vi "Get Model Construction - with check.vi"(1 "panel record":string[](array[string])) -> (0 "Fabric Array":string[][](array[string]))   [LabVIEW 2010]
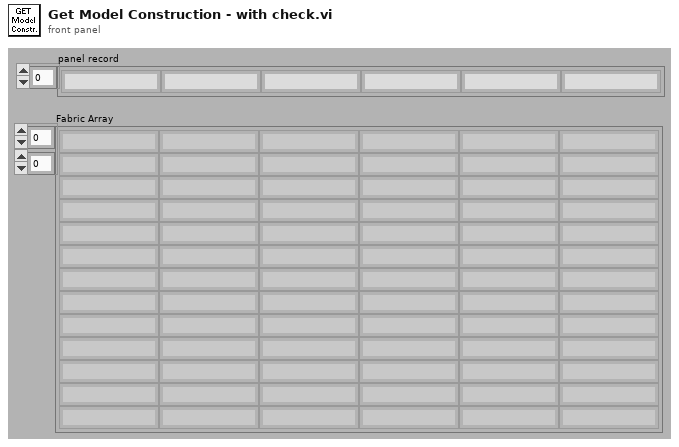
[diagram p1: front panel]
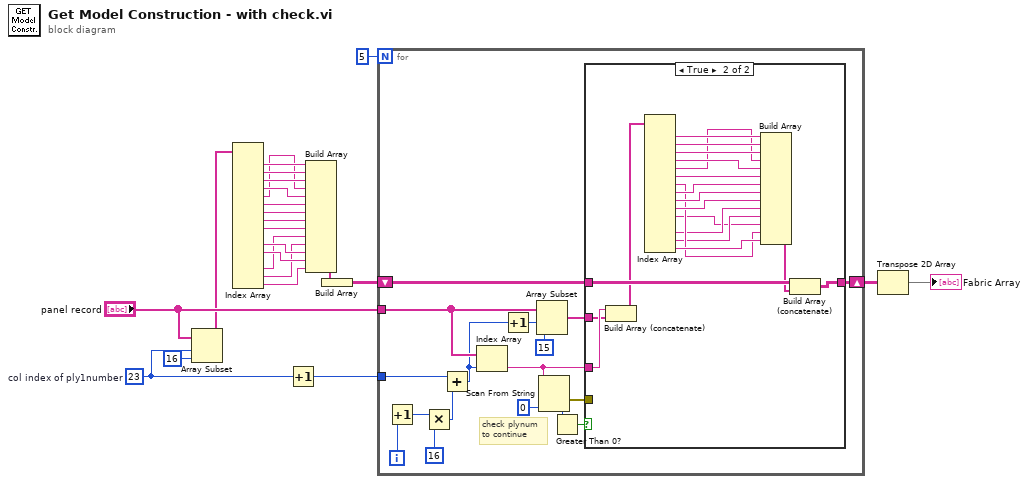
[diagram p0: block diagram]
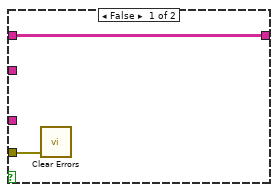
[diagram p2: hidden frame]
diagram:
  w23 = 23  # col index of ply1number
  n1 = Array Subset(array="panel record", index=w23, length=16) -> (w15:string[])
  n2 = Index Array(array=w15) -> (element #1=w7:string, element #2=w17:string, element #3=w16:string, element #4=w2:string, element #5=w1:string, element #6=w14:string, element #7=w13:string, element #8=w12:string, element #9=w11:string, element #11=w10:string, element #12=w9:string, element #14=w4:string, element #15=w5:string, element #16=w6:string)  [unwired: 16 in, 2 out]
  n3 = Increment(x=w23) -> (x+1=w3:i32)
  n4 = Build Array(w7, w17, w16, w1, w2, w14, w13, w12, w11, w4, w5, w10, w9, w6) -> (w8:string[])
  n5 = Build Array(w8) -> (w22:string[][])
  n6 = for {
    N: 5 -> [_]
    shift-right: [w38] -> w20
    shift-left: w22 -> [w39]
    tunnel: "panel record" -> [w32]
    tunnel: w3 -> [w37]
    i -> [w36]
    # "check plynum\nto continue"
    n7 = Increment(x=w36) -> (x+1=w33:i32)
    n8 = Multiply(x=w33, y=16) -> (x*y=w34:i32)
    n9 = Add(x=w37, y=w34) -> (x+y=w31:i32)
    n10 = Index Array(array=w32, index=w31) -> (element=w25:string)
    n11 = Increment(x=w31) -> (x+1=w29:i32)
    n12 = Array Subset(array=w32, index=w29, length=15) -> (w30:string[])
    n13 = Scan From String(input string=w25, default 1=i16 0 ("default value 1")) -> (error out=w26:errorcluster, output 1=w40:i16)  [unwired: 3 in, 2 out]
    n14 = Greater Than 0?(x=w40) -> (x > 0?=w41:bool)
    n15 = case shown="True" w41 {
      tunnel: [w43 w63] -> w38
      tunnel: w25 -> [_ w61]
      tunnel: w39 -> [w43 w62]
      tunnel: w30 -> [_ w60]
      tunnel: w26 -> [w42 _]
      frame False {
        n16 = call <vilib>:"Clear Errors.vi"("error in (no error)"=w42) -> ()  [unwired: 7 out]
      }
      frame True {
        n17 = Build Array (concatenate)(w61, w60) -> (w55:string[])
        n18 = Index Array(array=w55) -> (element #1=w59:string, element #2=w56:string, element #3=w57:string, element #4=w45:string, element #5=w44:string, element #6=w58:string, element #7=w49:string, element #8=w53:string, element #9=w52:string, element #10=w51:string, element #11=w46:string, element #13=w48:string, element #14=w47:string, element #15=w50:string)  [unwired: 15 in, 1 out]
        n19 = Build Array(w59, w56, w57, w44, w45, w58, w53, w52, w51, w48, w47, w46, w49, w50) -> (w54:string[])
        n20 = Build Array (concatenate)(w62, w54) -> (w63:string[][])
      }
    }
  }
  n21 = Transpose 2D Array(2D array=w20) -> (transposed array=→"Fabric Array":string[][])
